vi "consoleUi.vi"(8 "error in (no error)":errorcluster, 11 "Handler.UserEvent.Console in":refnum<class "Handler.UserEvent.Console.lvclass">) -> (0 "error out":errorcluster, 2 "Display User Event Logs":string, 3 "Handler.UserEvent.Console out":refnum<class "Handler.UserEvent.Console.lvclass">)   [LabVIEW 2017, in "Error Log.lvlib" / "Handler.UserEvent.Console.lvclass"]
uses:
  Handler.UserEvent.Console.lvclass
  \\192.168.1.40\Neosoft/Partage/Dossiers Personnels/BRO/DevTools_BR/wc/ErrorLog/src/Handler.UserEvent/Handler.UserEvent.lvclass
  \\192.168.1.40\Neosoft/Partage/Dossiers Personnels/BRO/DevTools_BR/wc/ErrorLog/src/Handler/Handler.lvclass
  Handler.UserEvent/Handler.UserEvent.lvclass/Handler.UserEvent.ctl
  Handler.UserEvent.Console.lvclass/Handler.UserEvent.Console.ctl
  Handler/Handler.lvclass/Handler.ctl
  Record/Record.lvclass/Record.ctl
  Record/Get Level.vi
  Handler.UserEvent/Get New Record.vi
  Get Private Events.vi
  Get Style Color.vi
  Handler/Get Caller VI Ref.vi
  Handler/Get Level.vi
  Record/Record.lvclass
panel:
  out "MsgLevel":string
  in  "Settings":bool
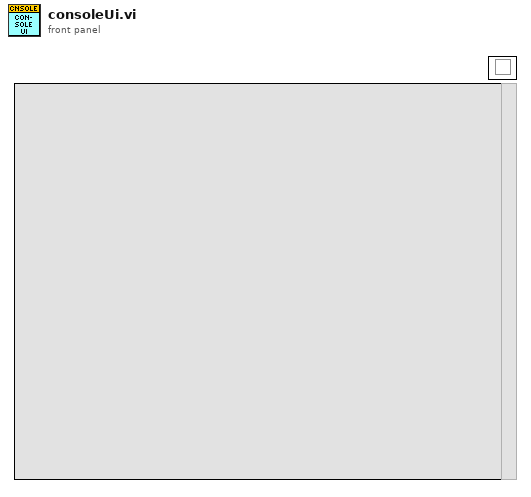
[diagram p1: front panel]
types:
  T1 = enum32{"Invalid", "Standard", "Closed", "Hidden", "Minimized", "Maximized"}
  T2 = typedef "Error Log.lvlib/Handler.UserEvent.Console.lvclass/privateEvents.ctl" = cluster{"Stop":refnum<user-event>, "Show Hide UI":refnum<user-event>, "Clear":refnum<user-event>}
  T3 = enum16{"DEBUG", "INFO", "WARNING", "ERROR", "CRITICAL"}
  T4 = cluster{"Public API:Properties:New Record":refnum<user-event>, "Public API:Properties:Private Events":T2}
  T5 = enum32{"Bad", "Idle", "Run top level", "Running"}
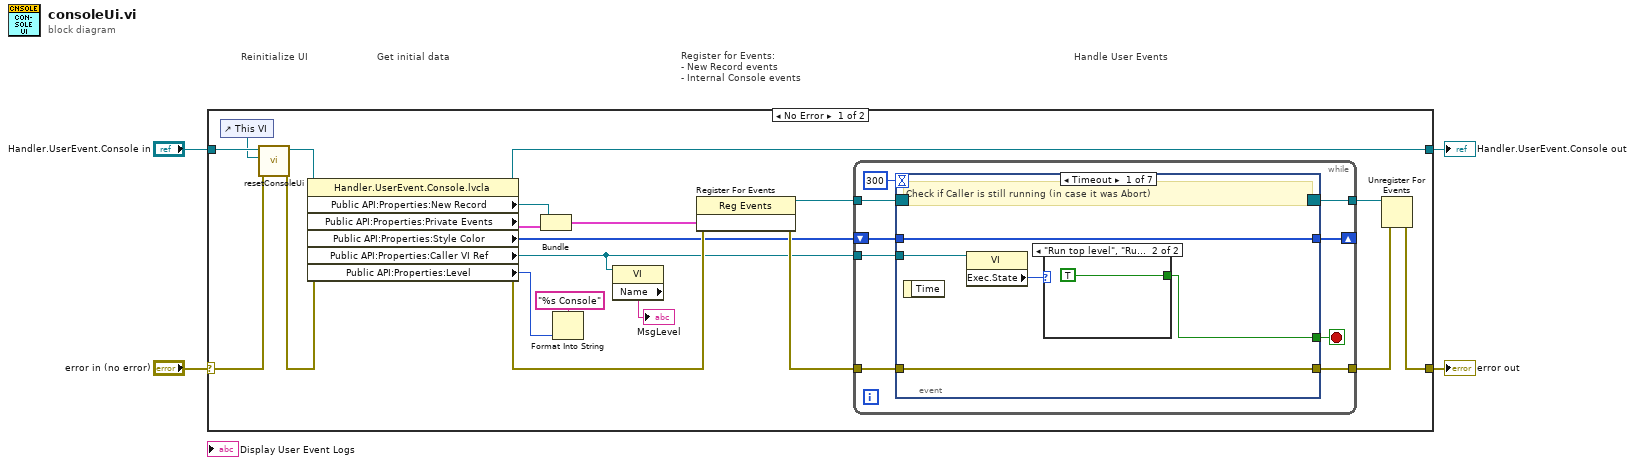
[diagram p0: block diagram]
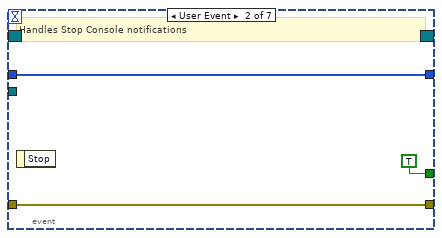
[diagram p3: hidden frame]
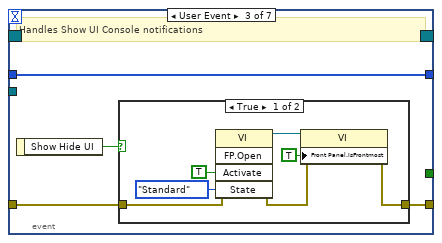
[diagram p4: hidden frame]
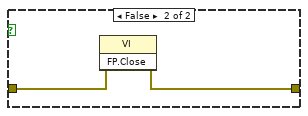
[diagram p5: hidden frame]
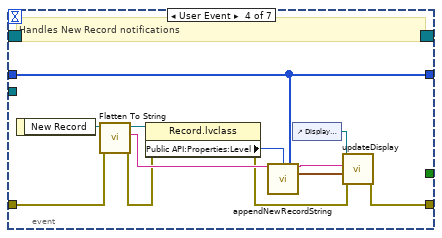
[diagram p6: hidden frame]
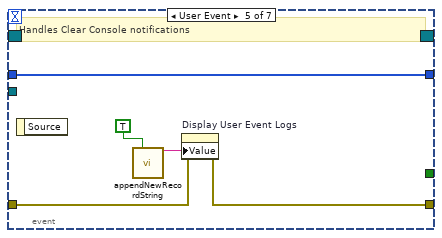
[diagram p7: hidden frame]
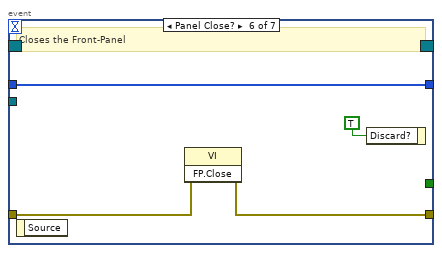
[diagram p8: hidden frame]
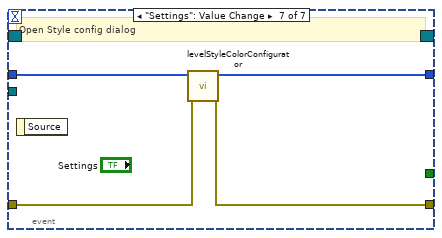
[diagram p9: hidden frame]
diagram:
  # "Handle User Events"
  # "Get initial data"
  # "Register for Events:\n- New Record events\n- Internal Console events"
  # "Reinitialize UI"
  n1 = case shown="No Error" "error in (no error)" {
    selector: "error in (no error)" -> [w13 w82]
    tunnel: [w18 w82] -> w3
    tunnel: [w16 w81] -> w1
    tunnel: "Handler.UserEvent.Console in" -> [w15 w81]
    frame No Error {
      n2 = control-ref of="This VI"() -> (w11:refnum<vi>)
      n3 = call "resetConsoleUi.vi"("error in (no error)"=w13, "reference"=w11, "Handler.UserEvent.Console in"=w15) -> ("error out"=w12:errorcluster, "Handler.UserEvent.Console out"=w14:refnum<class "Handler.UserEvent.Console.lvclass">)  [unwired: 7 in]
      n4 = property class="Handler.UserEvent.Console.lvcla"(reference=w14, error in=w12) -> (reference out=w16:refnum<class "Handler.UserEvent.Console.lvclass">, error out=w9:errorcluster, "Public API:Properties:New Record"=w24:refnum<user-event>, "Public API:Properties:Private Events"=w23:T2, "Public API:Properties:Style Color"=w8:u32[], "Public API:Properties:Caller VI Ref"=w6:refnum<vi>, "Public API:Properties:Level"=w7:T3)
      n5 = Bundle("Public API:Properties:New Record"=w24, "Public API:Properties:Private Events"=w23) -> (w22:T4)  [unwired: 1 in]
      n6 = Format Into String(format string="%s Console", w7) -> ()  [unwired: 2 in, 2 out]
      n7 = property class="VI"(reference=w6) -> ("Name"=→"MsgLevel":string)  [unwired: 1 in, 2 out]
      n8 = register-events(error in=w9, w22) -> (reference out=w21:refnum<event-registration>, error out=w17:errorcluster)  [unwired: 1 in]
      n9 = while {
        tunnel: w21 -> [w33]
        tunnel: w17 -> [w31]
        tunnel: [w30] -> w19
        tunnel: [w29] -> w20
        shift-right: [w28] -> _
        shift-left: w8 -> [w27]
        tunnel: w6 -> [w26]
        stop <- w32 stop-if-true
        n10 = event shown="[0] Timeout" {
          selector: w33 -> [_ _ _ _ _ _ _]
          dyn-events: [_ _ _ _ _ _ _] -> w29
          timeout: 300 -> [_ _ _ _ _ _ _]
          tunnel: [w34 TRUE _ _ _ _ _] -> w32
          tunnel: w31 -> [w38 w41 w45 w66 w72 w76 w78]
          tunnel: [w38 w41 w44 w58 w71 w75 w77] -> w30
          tunnel: [w37 w40 w43 w59 w68 w73 w80] -> w28
          tunnel: w27 -> [w37 w40 w43 w59 w68 w73 w79]
          tunnel: w26 -> [w36 _ _ _ _ _ _]
          event Timeout {
            # "Check if Caller is still running (in case it was Abort)"
            n11 = event-data() -> ()  [unwired: 1 in, 1 out]
            n12 = property class="VI"(reference=w36) -> ("Exec.State"=w35:T5)  [unwired: 1 in, 2 out]
            n13 = case shown="\"Run top level\", \"Running\"" w35 {
              tunnel: [_ TRUE] -> w34
              frame "Bad", Default {
              }
              frame "Run top level", "Running" {
              }
            }
          }
          event User Event {
            # "Handles Stop Console notifications"
            n14 = event-data() -> ()  [unwired: 1 in, 1 out]
          }
          event User Event {
            # "Handles Show UI Console notifications"
            n15 = event-data() -> ("Show Hide UI"=w46:bool)  [unwired: 1 in]
            n16 = case shown="True" w46 {
              tunnel: w45 -> [w51 w55]
              tunnel: [w47 w54] -> w44
              frame True {
                n17 = invoke class="VI" method="FP.Open"(error in=w51, "Activate"=TRUE ("Activate?"), "State"=T1."Standard") -> (reference out=w50:refnum<vi>, error out=w48:errorcluster)  [unwired: 2 in, 3 out]
                n18 = property class="VI"(reference=w50, error in=w48, "Front Panel.IsFrontmost"=TRUE ("Front Panel Window:Is Frontmost")) -> (error out=w47:errorcluster)  [unwired: 1 out]
              }
              frame False {
                n19 = invoke class="VI" method="FP.Close"(error in=w55) -> (error out=w54:errorcluster)  [unwired: 2 in, 2 out]
              }
            }
          }
          event User Event {
            # "Handles New Record notifications"
            n20 = event-data() -> ("New Record"=w67:refnum<class "Record.lvclass">)  [unwired: 1 in]
            n21 = call "Flatten To String.vi"("error in (no error)"=w66, "Record in"=w67) -> ("error out"=w57:errorcluster, "String"=w65:string, "Record out"=w64:refnum<class "Record.lvclass">)  [unwired: 7 in]
            n22 = property class="Record.lvclass"(reference=w64, error in=w57) -> (error out=w56:errorcluster, "Public API:Properties:Level"=w63:T3)  [unwired: 1 out]
            n23 = call "appendNewRecordString.vi"("New Record String"=w65, "Level"=w63, "Style Color"=w59) -> ("Log Display Updated"=w61:string, "Colors"=w62:cluster{"length":u32, "color":u32}[])  [unwired: 11 in]
            n24 = control-ref of="Display User Event Logs"() -> (w60:refnum<vi>)
            n25 = call "updateDisplay.vi"("error in (no error)"=w56, "Display Colors"=w62, "Log Display Updated"=w61, "reference"=w60) -> ("error out"=w58:errorcluster)  [unwired: 7 in]
          }
          event User Event {
            # "Handles Clear Console notifications"
            n26 = event-data() -> ()  [unwired: 1 in, 1 out]
            n27 = call "appendNewRecordString.vi"("clear"=TRUE) -> ("Log Display Updated"=w69:string)  [unwired: 13 in, 1 out]
            n28 = property on="Display User Event Logs" class="Str"(error in=w72, "Value"=w69) -> (error out=w71:errorcluster)  [unwired: 1 in, 1 out]
          }
          event Panel Close? {
            # "Closes the Front-Panel"
            n29 = event-data() -> ()  [unwired: 1 in, 1 out]
            n30 = invoke class="VI" method="FP.Close"(error in=w76) -> (error out=w75:errorcluster)  [unwired: 2 in, 2 out]
            n31 = event-data("Discard?"=TRUE) -> ()  [unwired: 1 in, 1 out]
          }
          event "Settings": Value Change {
            # "Open Style config dialog"
            n32 = event-data() -> ()  [unwired: 1 in, 1 out]
            n33 = call "levelStyleColorConfigurator.vi"("error in (no error)"=w78, "Colors in"=w79) -> ("error out"=w77:errorcluster, "Colors out"=w80:u32[])  [unwired: 8 in]
          }
        }
      }
      n34 = Unregister For Events(event registration refnum=w20, error in=w19) -> (error out=w18:errorcluster)
    }
    frame Error {
    }
  }
  "error out" <- w3
  "Handler.UserEvent.Console out" <- w1
